vi "add_to_ring_buffer.vi"(8 "error in":errorcluster, 9 "Buffer Position":i32, 10 "Ring Buffer":T1[](array[typedef]), 11 "Image":T1) -> (0 "error out":errorcluster, 1 "Buffer Image Out":T1, 2 "Ring Buffer Out":T1[](array[typedef]), 3 "Image Out":T1)   [LabVIEW 2016]
doc: "Adds image to specified place in IMAQ ring buffer."
uses:
  <vilib>/vision/Image Controls.llb/IMAQ Image.ctl
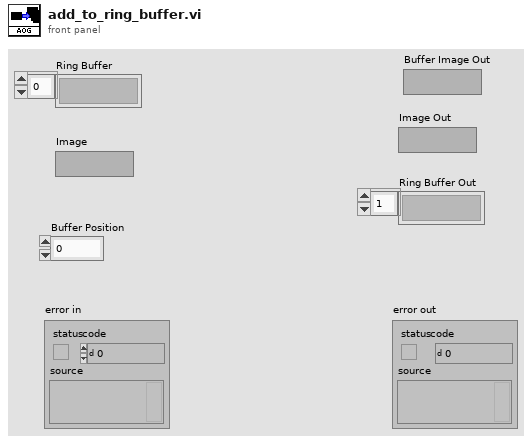
[diagram p1: front panel]
types:
  T1 = typedef "IMAQ Image.ctl" = refnum<image>
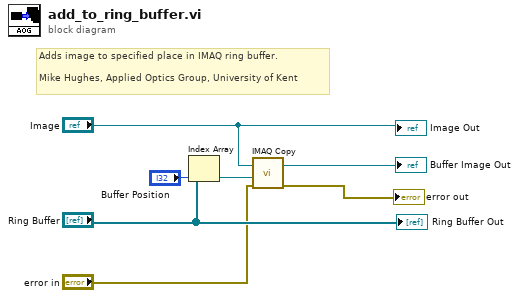
[diagram p0: block diagram]
diagram:
  # "Adds image to specified place in IMAQ ring buffer.\n\nMike Hughes, Applied Optics Group, University of Kent"
  n1 = Index Array(array="Ring Buffer", index="Buffer Position") -> (element=w6:T1)
  n2 = call "IMAQ Copy"("error in (no error)"="error in", "Image Dst"=w6, "Image Src"="Image") -> ("error out"=→"error out":errorcluster, "Image Dst Out"=→"Buffer Image Out":T1)  [unwired: 3 in]
  "Image Out" <- "Image"
  "Ring Buffer Out" <- "Ring Buffer"
